vi "通信并与其他模块交互 (子VI).vi"() -> ()   [LabVIEW 2016, in "质控单元.lvlib"]
uses:
  <vilib>/Plasmionique/MB Master/MB_Master_TCP/MB_Master_TCP.lvclass
  D:/Program Files (x86)/National Instruments/LabVIEW 2016/vi.lib/Plasmionique/MB Master/MB_Master/MB_Master.lvclass
  <vilib>/Plasmionique/MB Master/MB_Master/MB_Master.lvclass
  <vilib>/Plasmionique/MB Master/MB Master.lvlib
  <vilib>/Utility/config.llb/NI_LVConfig.lvlib
panel:
  out "CODCr测量状态":u16[](array[numeric])
  out "CODMn测量状态":u16[](array[numeric])
  out "总氮测量状态":u16[](array[numeric])
  out "总磷测量状态":u16[](array[numeric])
  out "氨氮测量状态":u16[](array[numeric])
  out "通讯状态":bool
  out "待处理插入数量":i32
  out "元素":cluster{"命令":string}[](array[cluster])
  out "队列中元素数量":i32
  in  "starting address 6":u16
  in  "values 6":u16[](array[numeric])
  in  "starting address 5":u16
  in  "values 5":u16[](array[numeric])
  in  "starting address 4":u16
  in  "values 4":u16[](array[numeric])
  in  "starting address 3":u16
  in  "values 3":u16[](array[numeric])
  in  "starting address 2":u16
  in  "values 2":u16[](array[numeric])
  in  "values":u16[](array[numeric])
  in  "starting address":u16
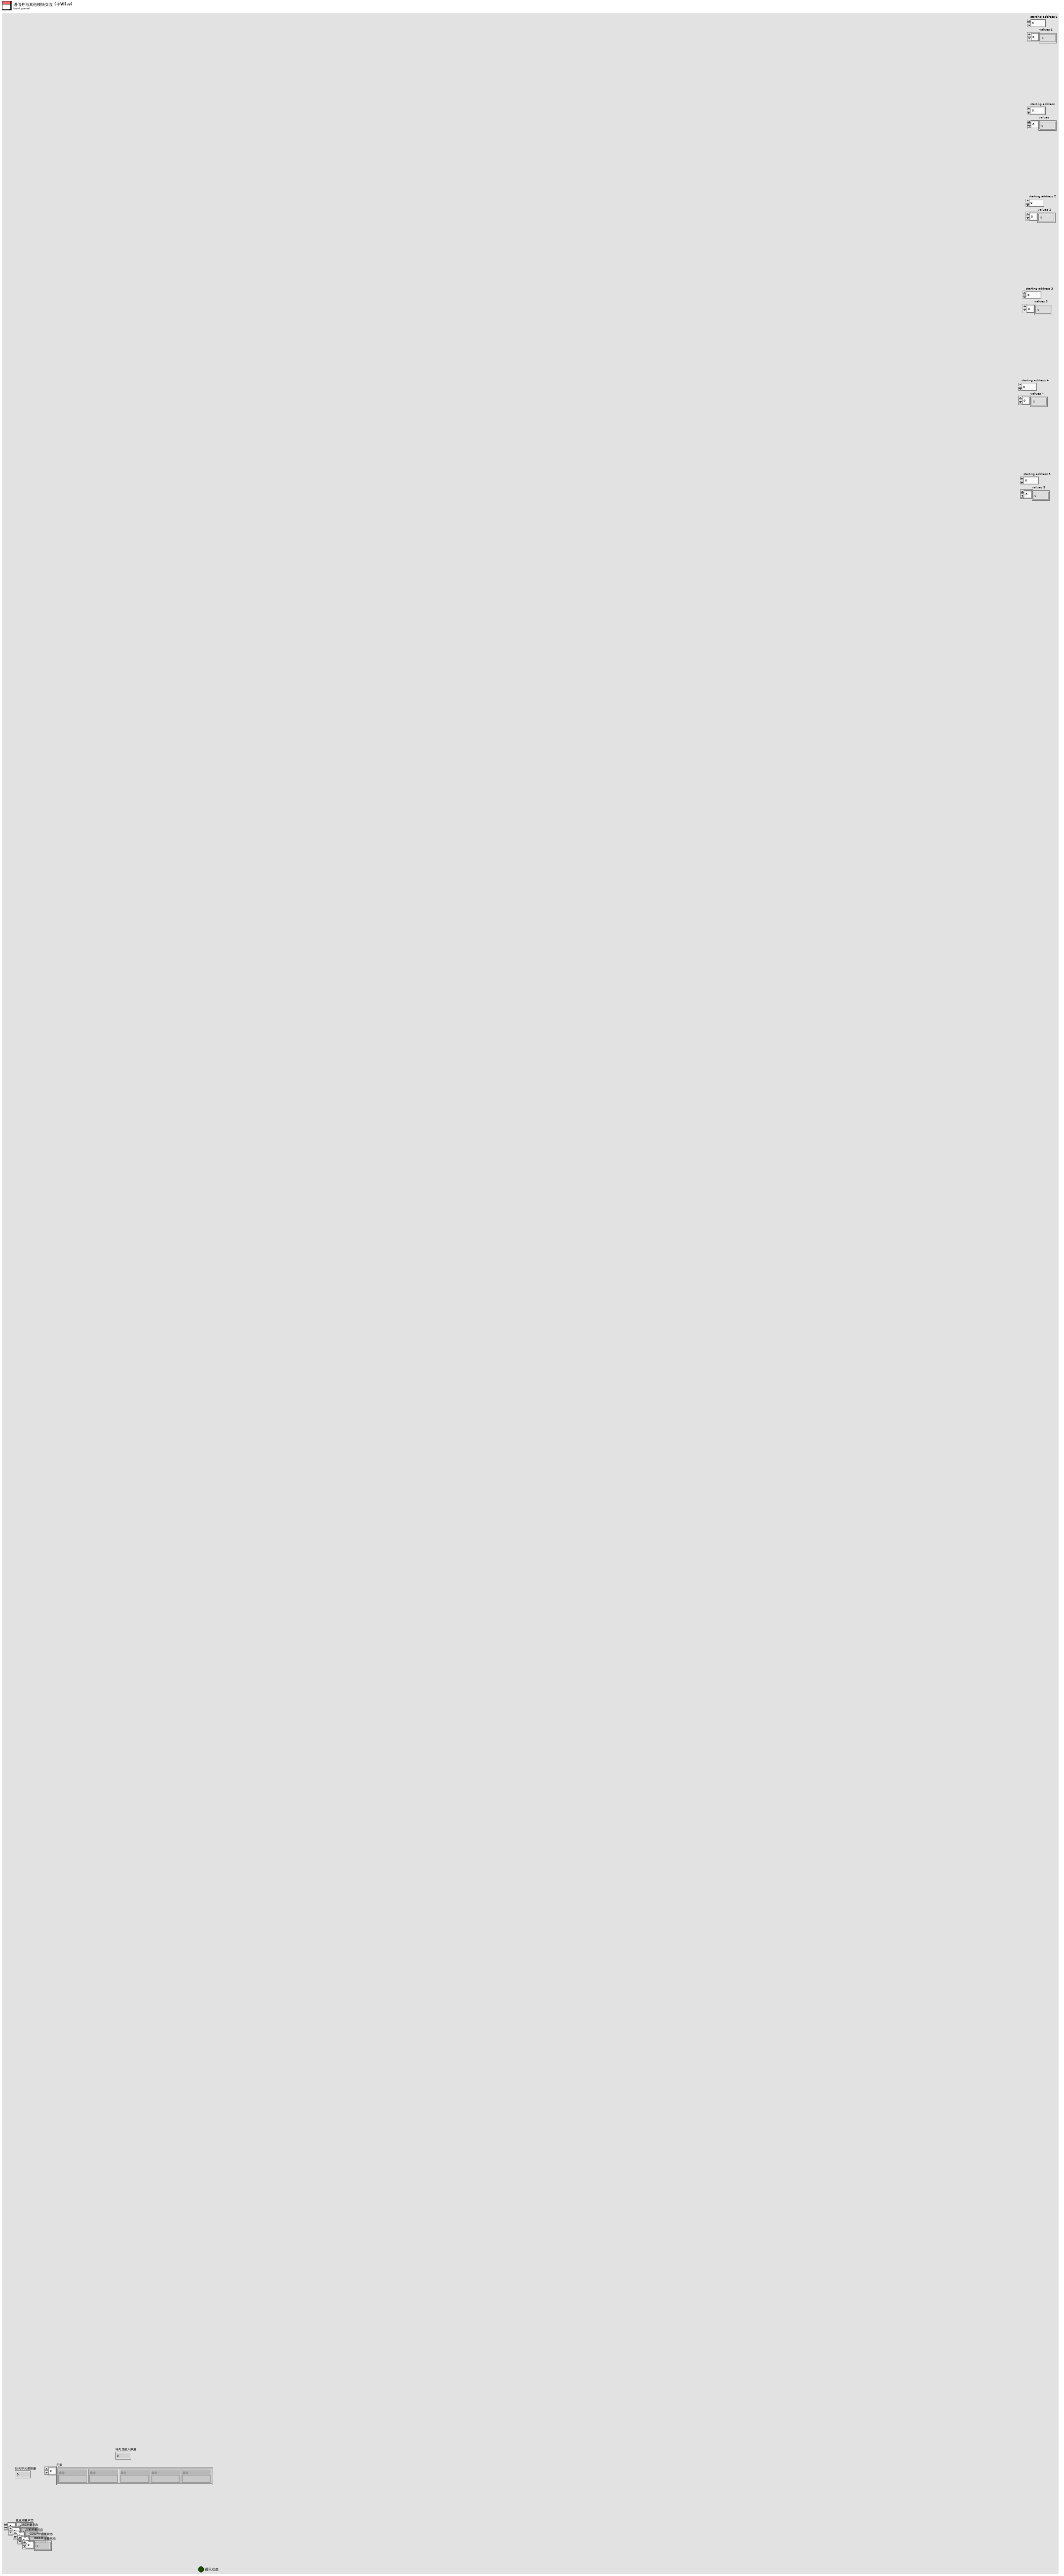
[diagram p1: front panel]
types:
  T1 = typedef "NI_LVConfig.lvlib/Config Data RefNum.ctl" = refnum<k1>
  T2 = cluster{"因子编码":u32, "单位":u16, "标样参考值":sgl, "水样数据时间":timestamp, "水样实测值":sgl, "水样数据标识":string, "标样数据时间":timestamp, "标样实测值":sgl, "标样数据标识":string, "空白数据时间":timestamp, "空白实测值":sgl, "空白数据标识":string, "零点核查数据时间":timestamp, "零点核查实测值":sgl, "零点核查数据标识":string, "跨度核查数据时间":timestamp, "跨度核查实测值":sgl, "跨度核查数据标识":string, "加标回收数据时间":timestamp, "加标回收实测值":sgl, "加标回收数据标识":string, "平行样数据时间":timestamp, "平行样实测值":sgl, "平行样数据标识":string}
  T3 = cluster{"系统时间":timestamp, "工作状态":enum16{"空闲", "水样测试", "标样核查", "零点核查", "跨度核查", "空白测试", "平行样测试", "加标回收", "空白校准", "标样校准", "初始化（清洗）"}, "测量模式":enum16{"待机", "连续模式", "周期模式", "定点模式", "受控模式", "手动模式"}, "告警代码":enum16{"无告警", "缺试剂告警", "缺水样告警", "缺蒸馏水告警", "缺标液告警", "仪表漏液告警", "标定异常告警", "超量程告警", "加热异常", "低试剂预警", "超上限告警", "超下限告警", "仪表内部其他异常", "滴定异常告警", "电极异常告警", "量程切换告警", "参数设置告警", "PH电极电位异常", "电导率电极异常", "浊度光度异常", "溶解氧电极异常", "溶解氧光强异常", "温度异常告警", "PH异常告警", "溶解氧异常告警", "电导率异常告警", "浊度异常告警", "叶绿素异常告警", "藻密度异常告警", "蓝绿藻异常告警", "ORP异常告警", "氨氮异常告警", "清洁刷异常告警", "SD卡异常告警", "蓝牙异常告警", "Wifi异常告警", "流程异常告警"}, "故障代码":enum16{"无故障", "电机故障", "温度故障", "通讯故障", "滴定故障"}, "日志代码":u16, "软件版本":u16, "F0":sgl, "F1":sgl, "F2":sgl, "F3":sgl, "T":sgl, "H":sgl, "id":u16, "flowid":u16, "量程":u16, "总磷控温温度1":sgl, "营养盐控温温度2":sgl, "ADC":sgl}
  T4 = cluster{"Registers[0]":u16, "Registers[1]":u16, "Registers[2]":u16, "Registers[3]":u16, "Registers[4]":u16, "Registers[5]":u16, "Registers[6]":u16, "Registers[7]":u16, "Registers[8]":u16, "Registers[9]":u16, "Registers[10]":u16, "Registers[11]":u16, "Registers[12]":u16, "Registers[13]":u16, "Registers[14]":u16, "Registers[15]":u16, "Registers[16]":u16, "Registers[17]":u16, "Registers[18]":u16, "Registers[19]":u16, "Registers[20]":u16, "Registers[21]":u16, "Registers[22]":u16, "Registers[23]":u16, "Registers[24]":u16, "Registers[25]":u16, "Registers[26]":u16, "Registers[27]":u16, "Registers[28]":u16, "Registers[29]":u16, "Registers[30]":u16, "Registers[31]":u16, "Registers[32]":u16, "Registers[33]":u16, "Registers[34]":u16, "Registers[35]":u16, "Registers[36]":u16, "Registers[37]":u16, "Registers[38]":u16, "Registers[39]":u16, "Registers[40]":u16, "Registers[41]":u16, "Registers[42]":u16, "Registers[43]":u16, "Registers[44]":u16, "Registers[45]":u16, "Registers[46]":u16, "Registers[47]":u16, "Registers[48]":u16, "Registers[49]":u16, "Registers[50]":u16, "Registers[51]":u16, "Registers[52]":u16, "Registers[53]":u16, "Registers[54]":u16, "Registers[55]":u16, "Registers[56]":u16}
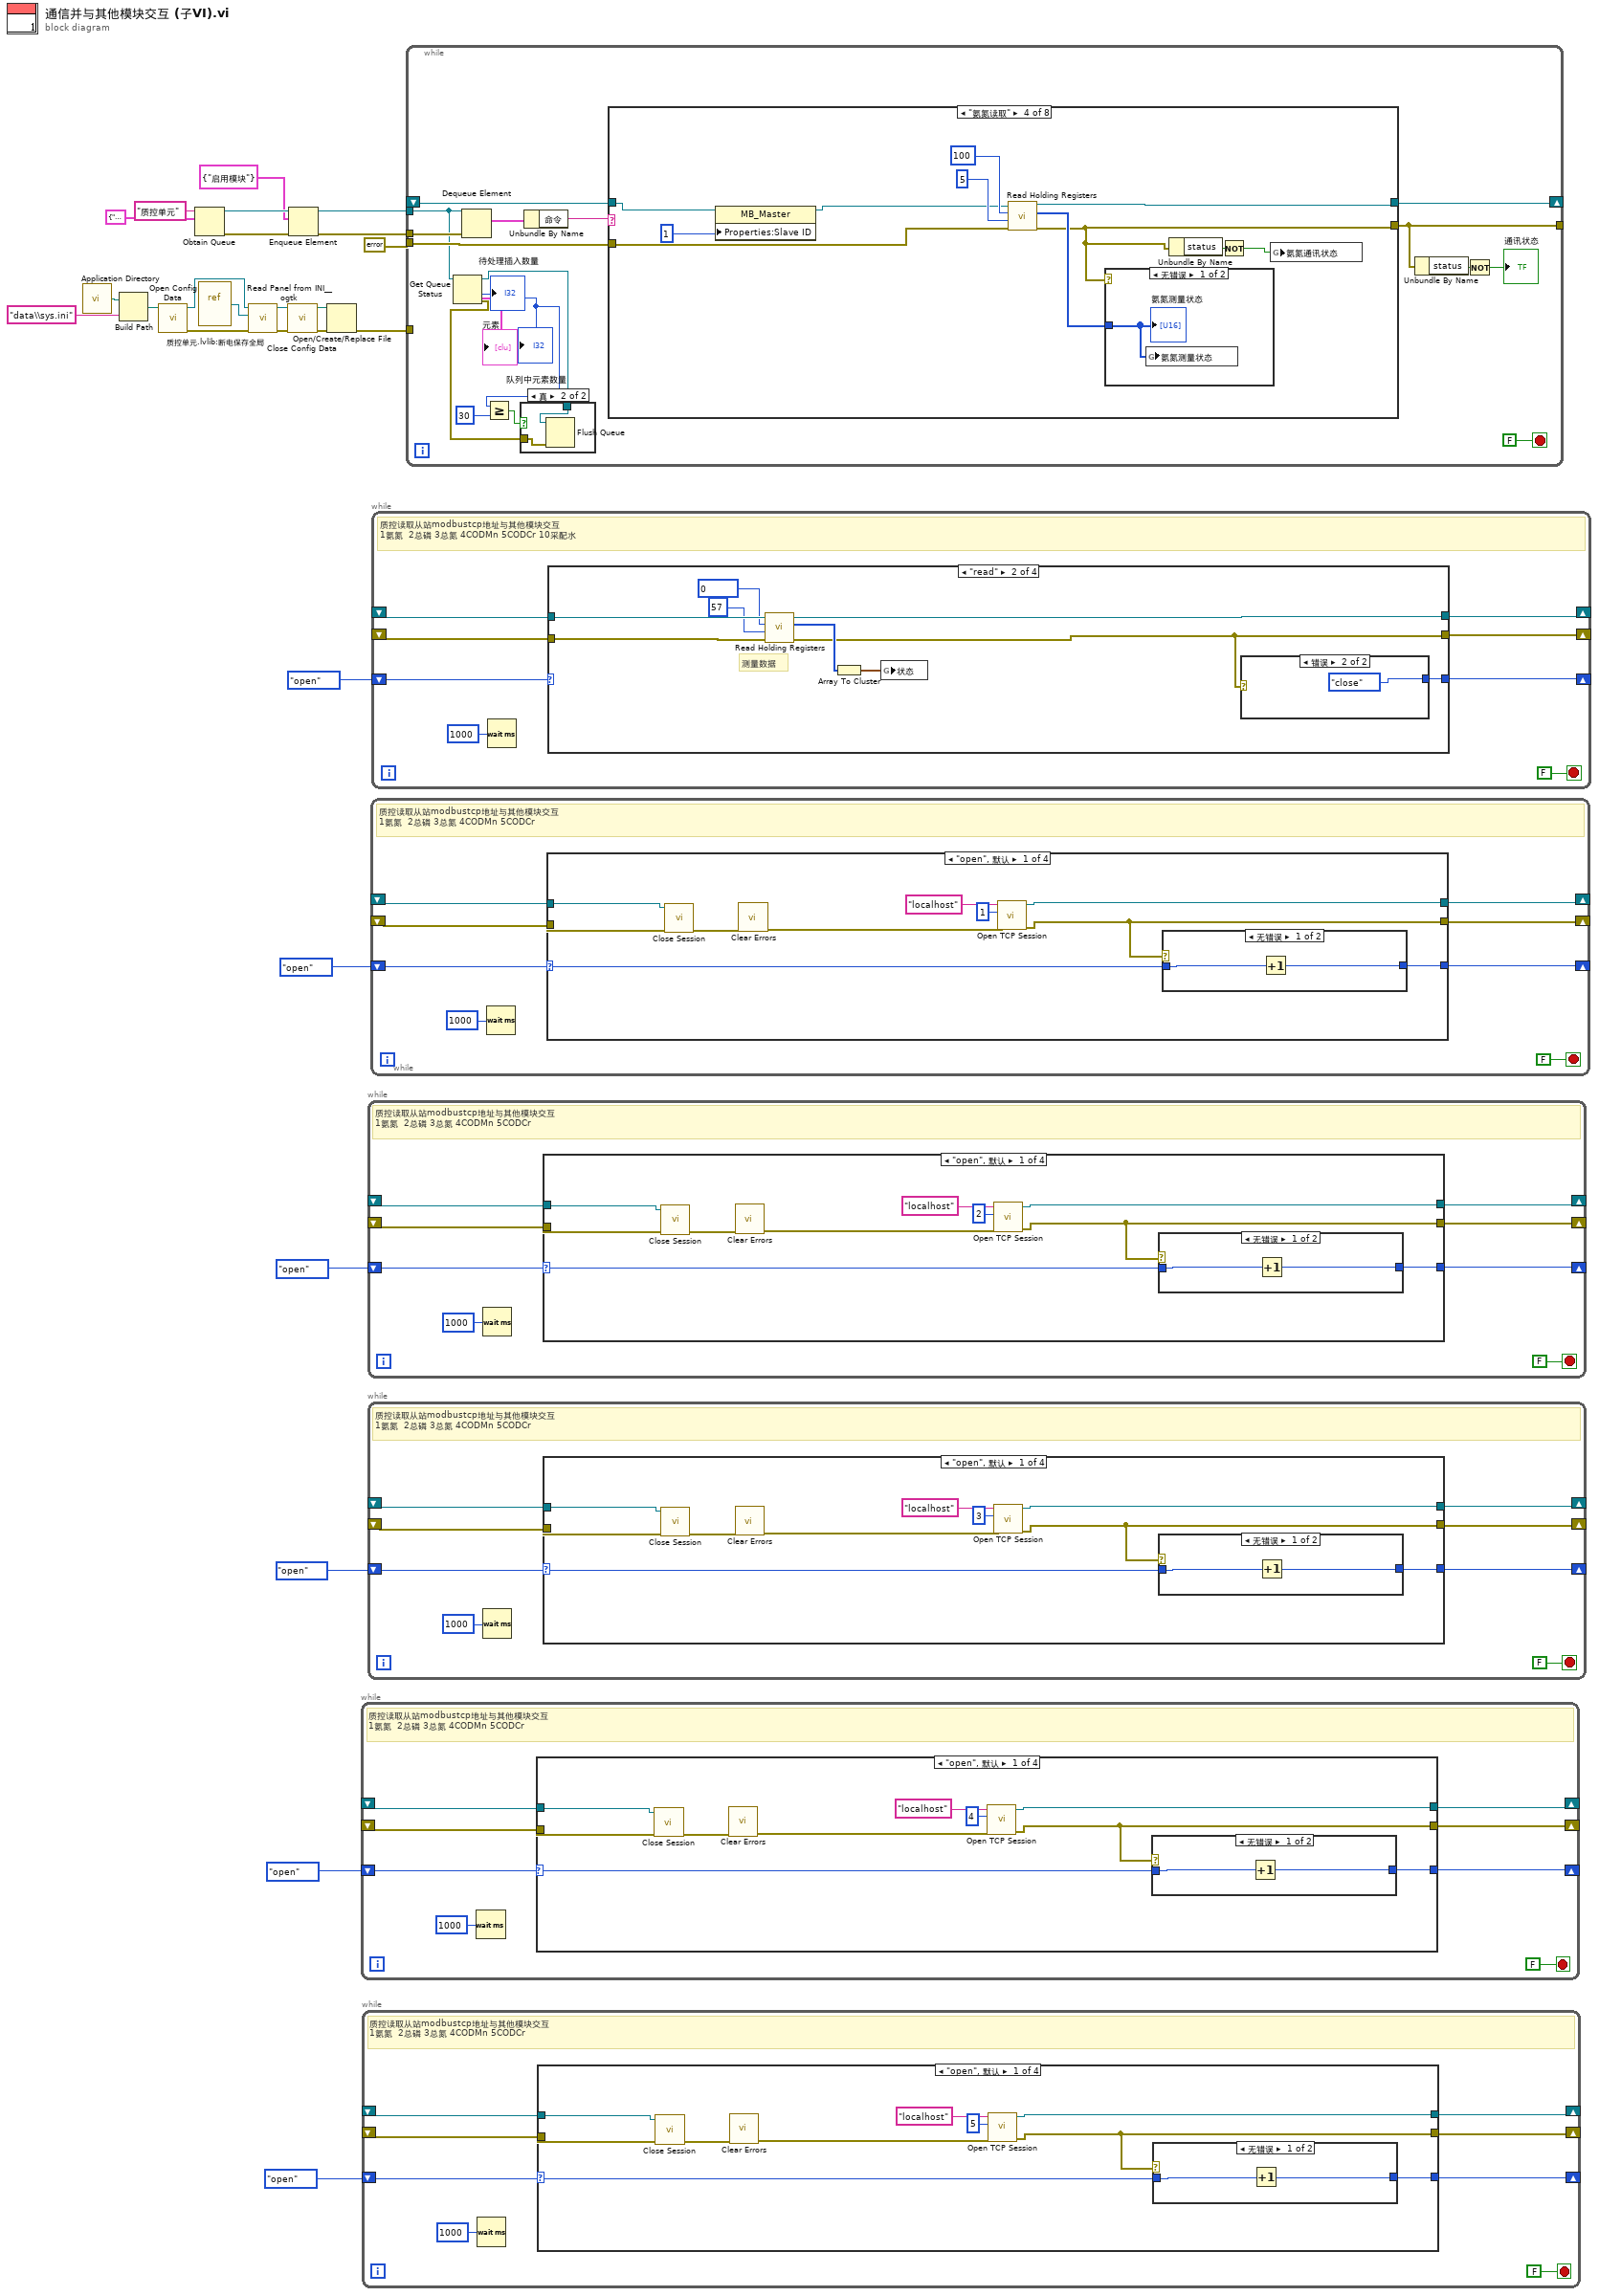
[diagram p0: block diagram]
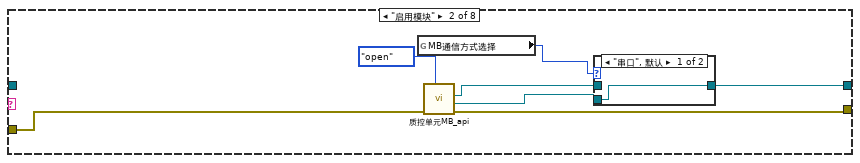
[diagram p4: hidden frame]
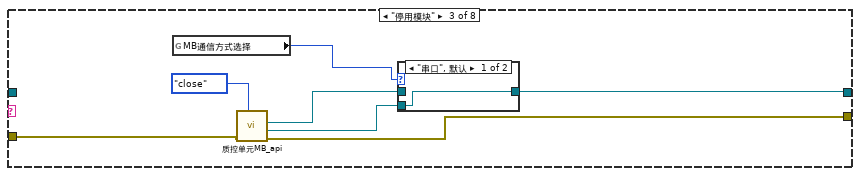
[diagram p6: hidden frame]
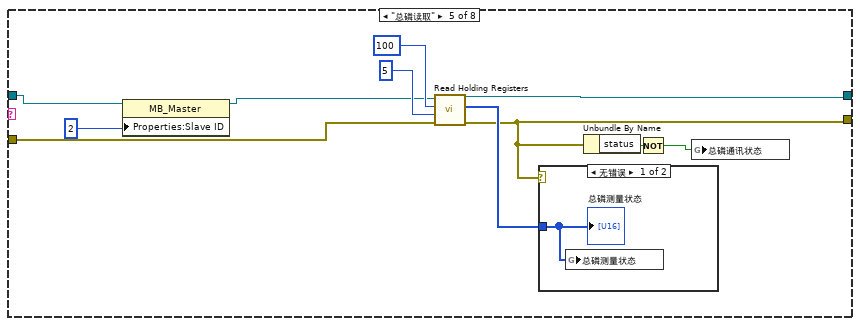
[diagram p9: hidden frame]
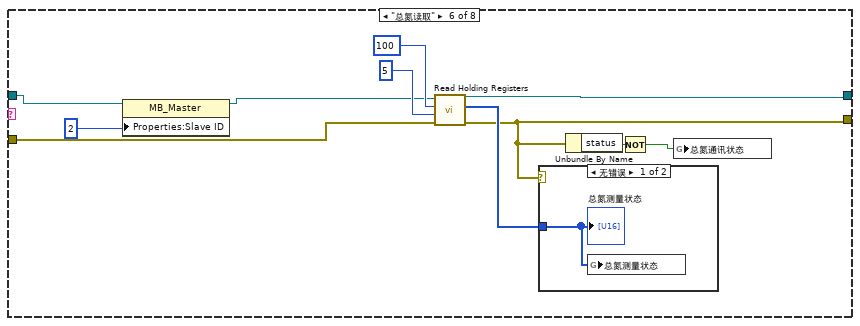
[diagram p11: hidden frame]
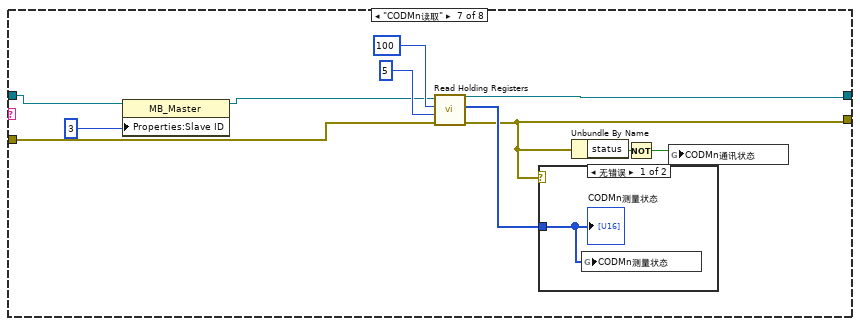
[diagram p13: hidden frame]
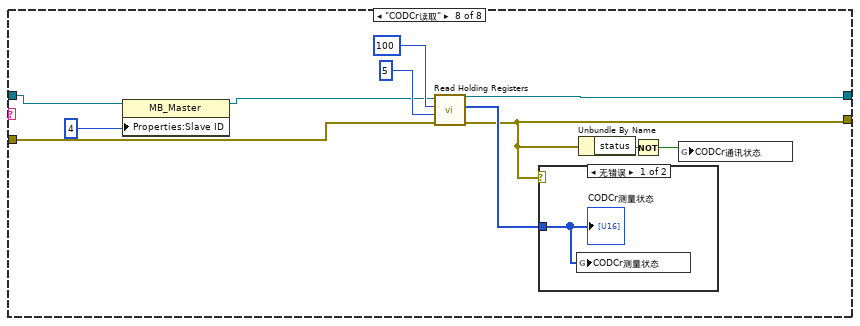
[diagram p15: hidden frame]
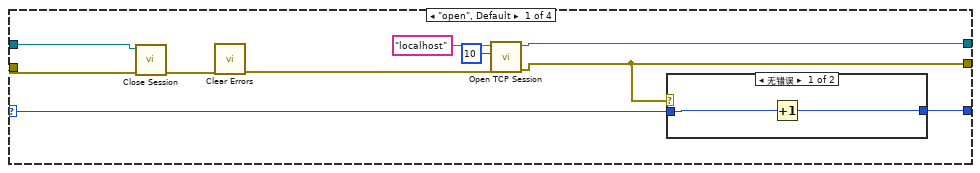
[diagram p17: hidden frame]
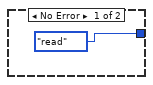
[diagram p19: hidden frame]
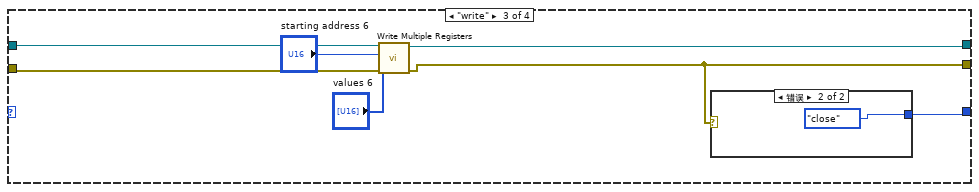
[diagram p20: hidden frame]
diagram:
  n1 = call <vilib>:"Application Directory.vi"() -> ("Application Directory"=w13:path)
  n2 = Build Path(base path=w13, name or relative path="data\\sys.ini" ("名称或相对路径")) -> (appended path=w11:path)
  n3 = call <vilib>:"Open Config Data.vi"("configuration file path"=w11) -> ("error out"=w7:errorcluster, "refnum"=w10:T1)  [unwired: 8 in, 1 out]
  n4 = Obtain Queue(name (unnamed)="质控单元" ("名称（未命名）"), element data type=cluster{"命令":string} {"命令"="启用模块"} ("元素")) -> (queue out=w16:refnum<queue>, error out=w15:errorcluster)  [unwired: 3 in, 1 out]
  n5 = vi-ref "质控单元.lvlib:断电保存全局.vi"() -> (w9:refnum<vi>)
  n6 = call <userlib>:"Read Panel from INI__ogtk.vi"("error in (no error)"=w7, "VI ref"=w9, "refnum"=w10) -> ("error out"=w6:errorcluster, "refnum out"=w8:T1)  [unwired: 7 in]
  n7 = call <vilib>:"Close Config Data.vi"("error in (no error)"=w6, "refnum"=w8) -> ("error out"=w5:errorcluster, "file path"=w4:path)  [unwired: 8 in]
  n8 = Enqueue Element(queue=w16, element=cluster{"命令":string} {"命令"="启用模块"} ("元素"), error in (no error)=w15) -> (queue out=w2:refnum<queue>, error out=w1:errorcluster)  [unwired: 1 in, 1 out]
  n9 = Open/Create/Replace File(file path (use dialog)=w4, error in=w5) -> (error out=w3:errorcluster)  [unwired: 4 in, 2 out]
  n10 = while {
    shift-right: [w31] -> _
    shift-left: _ -> [w33]
    shift-right: [w30] -> _
    shift-left: _ -> [w32]
    shift-right: [w27] -> _
    shift-left: enum16{"open", "read", "write", "close"}."open" -> [w28]
    stop <- FALSE stop-if-true
    # "质控读取从站modbustcp地址与其他模块交互\n1氨氮  2总磷 3总氮 4CODMn 5CODCr"
    n11 = Wait (ms)(milliseconds to wait=u32 1000 ("等待时间（毫秒）")) -> ()  [unwired: 1 out]
    n12 = case shown="\"open\", 默认" w28 {
      selector: w28 -> [w35 _ _ _]
      tunnel: w33 -> [w40 w71 w79 w87]
      tunnel: w32 -> [w39 w68 w78 w86]
      tunnel: [w41 w66 w77 w87] -> w31
      tunnel: [w36 w65 w76 w84] -> w30
      tunnel: [w34 w67 w80 enum16{"open", "read", "write", "close"}."open"] -> w27
      frame "open", Default {
        n13 = call-dynamic "Close Session.vi"("error in (no error)"=w39, "MB session in"=w40) -> ("error out"=w38:errorcluster)  [unwired: 9 in]
        n14 = call <vilib>:"Clear Errors.vi"("error in (no error)"=w38) -> ("error out"=w37:errorcluster)  [unwired: 5 in, 1 out]
        n15 = call <vilib>:"Open TCP Session.vi"("error in (no error)"=w37, "Port (502)"=u16 4, "IP Address"="localhost") -> ("error out"=w36:errorcluster, "MB_TCP session"=w41:refnum<class "MB_Master_TCP.lvclass">)  [unwired: 7 in]
        n16 = case shown="无错误" w36 {
          tunnel: w35 -> [w45 w46]
          tunnel: [w44 w46] -> w34
          frame No Error {
            n17 = Increment(x=w45) -> (x+1=w44:enum16{"open", "read", "write", "close"})
          }
          frame Error {
          }
        }
      }
      frame "read" {
        # "测量数据"
        n18 = call <vilib>:"Read Holding Registers.vi"("error in (no error)"=w68, "quantity"=u16 30, "starting address"=u16 0, "MB session in"=w71) -> ("error out"=w65:errorcluster, "Registers"=w64:u16[], "MB session out"=w66:refnum<class "MB_Master.lvclass">)  [unwired: 5 in]
        n19 = Index Array(array=w64) -> (element #1=w63:u16, element #2=w62:u16, element #3=w61:u16, element #4=w57:u16, element #5=w56:u16, element #6=w55:u16, element #7=w54:u16, element #8=w52:u16, element #9=w51:u16, element #10=w50:u16)  [unwired: 10 in]
        n20 = Build Array(w62, w61) -> (w60:u16[])
        n21 = Build Array(w56, w55, w54, w52, w51, w50) -> (w53:u16[])
        n22 = call "HexToDate.vi"("数组"=w53) -> ("DATE"=w49:timestamp[])  [unwired: 10 in]
        n23 = call "HexToCDABFloat.vi"("数组"=w60) -> ("FLOAT"=w59:sgl[])  [unwired: 10 in]
        n24 = Index Array(array=w49) -> (element #1=w48:timestamp, element #2=w47:timestamp)  [unwired: 2 in]
        n25 = Index Array(array=w59) -> (element=w58:sgl)  [unwired: 1 in]
        n26 = global write "与CODMn交互全局.vi" "COD浓度（mg/L)"(w58) -> ()
        n27 = global write "与CODMn交互全局.vi" "加标回收启动时间"(w48) -> ()
        n28 = global write "与CODMn交互全局.vi" "CODMn工作状态"(w63) -> ()
        n29 = global write "与CODMn交互全局.vi" "水样启动时间"(w47) -> ()
        n30 = global write "与CODMn交互全局.vi" "多列列表框"(w57) -> ()
        n31 = case shown="错误" w65 {
          tunnel: [enum16{"open", "read", "write", "close"}."read" enum16{"open", "read", "write", "close"}."close"] -> w67
          frame No Error {
          }
          frame Error {
          }
        }
      }
      frame "write" {
        n32 = call <vilib>:"Write Multiple Registers.vi"("error in (no error)"=w78, "values"="values 4", "starting address"="starting address 4", "MB session in"=w79) -> ("error out"=w76:errorcluster, "MB session out"=w77:refnum<class "MB_Master.lvclass">)  [unwired: 6 in]
        n33 = case shown="错误" w76 {
          tunnel: [enum16{"open", "read", "write", "close"}."read" enum16{"open", "read", "write", "close"}."close"] -> w80
          frame No Error {
          }
          frame Error {
          }
        }
      }
      frame "close" {
        n34 = call-dynamic "Close Session.vi"("error in (no error)"=w86, "MB session in"=w87) -> ("error out"=w85:errorcluster)  [unwired: 9 in]
        n35 = call <vilib>:"Clear Errors.vi"("error in (no error)"=w85) -> ("error out"=w84:errorcluster)  [unwired: 5 in, 1 out]
      }
    }
  }
  n36 = while {
    shift-right: [w93] -> _
    shift-left: _ -> [w95]
    shift-right: [w92] -> _
    shift-left: _ -> [w94]
    shift-right: [w89] -> _
    shift-left: enum16{"open", "read", "write", "close"}."open" -> [w90]
    stop <- FALSE stop-if-true
    # "质控读取从站modbustcp地址与其他模块交互\n1氨氮  2总磷 3总氮 4CODMn 5CODCr"
    n37 = Wait (ms)(milliseconds to wait=u32 1000 ("等待时间（毫秒）")) -> ()  [unwired: 1 out]
    n38 = case shown="\"open\", 默认" w90 {
      selector: w90 -> [w97 _ _ _]
      tunnel: w95 -> [w102 w123 w131 w139]
      tunnel: w94 -> [w101 w120 w130 w138]
      tunnel: [w103 w114 w129 w139] -> w93
      tunnel: [w98 w113 w128 w136] -> w92
      tunnel: [w96 w119 w132 enum16{"open", "read", "write", "close"}."open"] -> w89
      frame "open", Default {
        n39 = call-dynamic "Close Session.vi"("error in (no error)"=w101, "MB session in"=w102) -> ("error out"=w100:errorcluster)  [unwired: 9 in]
        n40 = call <vilib>:"Clear Errors.vi"("error in (no error)"=w100) -> ("error out"=w99:errorcluster)  [unwired: 5 in, 1 out]
        n41 = call <vilib>:"Open TCP Session.vi"("error in (no error)"=w99, "Port (502)"=u16 5, "IP Address"="localhost") -> ("error out"=w98:errorcluster, "MB_TCP session"=w103:refnum<class "MB_Master_TCP.lvclass">)  [unwired: 7 in]
        n42 = case shown="无错误" w98 {
          tunnel: w97 -> [w107 w108]
          tunnel: [w106 w108] -> w96
          frame No Error {
            n43 = Increment(x=w107) -> (x+1=w106:enum16{"open", "read", "write", "close"})
          }
          frame Error {
          }
        }
      }
      frame "read" {
        # "状态告警"
        # "测量数据"
        n44 = call <vilib>:"Read Holding Registers.vi"("error in (no error)"=w120, "quantity"=u16 83, "starting address"=u16 4096, "MB session in"=w123) -> ("error out"=w115:errorcluster, "Registers"=w112:u16[], "MB session out"=w116:refnum<class "MB_Master.lvclass">)  [unwired: 5 in]
        n45 = call "交互测量数据区解析.vi"("数组"=w112) -> ("测量数据区"=w110:T2)  [unwired: 10 in]
        n46 = global write "与CODCr交互全局.vi" "CODCr测量数据区"(w110) -> ()
        n47 = call <vilib>:"Read Holding Registers.vi"("error in (no error)"=w115, "quantity"=u16 24, "starting address"=u16 4224, "MB session in"=w116) -> ("error out"=w113:errorcluster, "Registers"=w111:u16[], "MB session out"=w114:refnum<class "MB_Master.lvclass">)  [unwired: 5 in]
        n48 = call "交互状态告警区解析.vi"("数组"=w111) -> ("状态告警区"=w109:T3)  [unwired: 10 in]
        n49 = global write "与CODCr交互全局.vi" "CODCr状态告警区"(w109) -> ()
        n50 = case shown="错误" w113 {
          tunnel: [enum16{"open", "read", "write", "close"}."read" enum16{"open", "read", "write", "close"}."close"] -> w119
          frame No Error {
          }
          frame Error {
          }
        }
      }
      frame "write" {
        n51 = call <vilib>:"Write Multiple Registers.vi"("error in (no error)"=w130, "values"="values 5", "starting address"="starting address 5", "MB session in"=w131) -> ("error out"=w128:errorcluster, "MB session out"=w129:refnum<class "MB_Master.lvclass">)  [unwired: 6 in]
        n52 = case shown="错误" w128 {
          tunnel: [enum16{"open", "read", "write", "close"}."read" enum16{"open", "read", "write", "close"}."close"] -> w132
          frame No Error {
          }
          frame Error {
          }
        }
      }
      frame "close" {
        n53 = call-dynamic "Close Session.vi"("error in (no error)"=w138, "MB session in"=w139) -> ("error out"=w137:errorcluster)  [unwired: 9 in]
        n54 = call <vilib>:"Clear Errors.vi"("error in (no error)"=w137) -> ("error out"=w136:errorcluster)  [unwired: 5 in, 1 out]
      }
    }
  }
  n55 = while {
    shift-right: [w145] -> _
    shift-left: _ -> [w147]
    shift-right: [w144] -> _
    shift-left: _ -> [w146]
    shift-right: [w141] -> _
    shift-left: enum16{"open", "read", "write", "close"}."open" -> [w142]
    stop <- FALSE stop-if-true
    # "质控读取从站modbustcp地址与其他模块交互\n1氨氮  2总磷 3总氮 4CODMn 5CODCr"
    n56 = Wait (ms)(milliseconds to wait=u32 1000 ("等待时间（毫秒）")) -> ()  [unwired: 1 out]
    n57 = case shown="\"open\", 默认" w142 {
      selector: w142 -> [w149 _ _ _]
      tunnel: w147 -> [w154 w175 w183 w191]
      tunnel: w146 -> [w153 w172 w182 w190]
      tunnel: [w155 w166 w181 w191] -> w145
      tunnel: [w150 w165 w180 w188] -> w144
      tunnel: [w148 w171 w184 enum16{"open", "read", "write", "close"}."open"] -> w141
      frame "open", Default {
        n58 = call-dynamic "Close Session.vi"("error in (no error)"=w153, "MB session in"=w154) -> ("error out"=w152:errorcluster)  [unwired: 9 in]
        n59 = call <vilib>:"Clear Errors.vi"("error in (no error)"=w152) -> ("error out"=w151:errorcluster)  [unwired: 5 in, 1 out]
        n60 = call <vilib>:"Open TCP Session.vi"("error in (no error)"=w151, "Port (502)"=u16 2, "IP Address"="localhost") -> ("error out"=w150:errorcluster, "MB_TCP session"=w155:refnum<class "MB_Master_TCP.lvclass">)  [unwired: 7 in]
        n61 = case shown="无错误" w150 {
          tunnel: w149 -> [w159 w160]
          tunnel: [w158 w160] -> w148
          frame No Error {
            n62 = Increment(x=w159) -> (x+1=w158:enum16{"open", "read", "write", "close"})
          }
          frame Error {
          }
        }
      }
      frame "read" {
        # "状态告警"
        # "测量数据"
        n63 = call <vilib>:"Read Holding Registers.vi"("error in (no error)"=w172, "quantity"=u16 83, "starting address"=u16 4096, "MB session in"=w175) -> ("error out"=w167:errorcluster, "Registers"=w164:u16[], "MB session out"=w168:refnum<class "MB_Master.lvclass">)  [unwired: 5 in]
        n64 = call "交互测量数据区解析.vi"("数组"=w164) -> ("测量数据区"=w162:T2)  [unwired: 10 in]
        n65 = global write "与总磷交互全局.vi" "总磷测量数据区"(w162) -> ()
        n66 = call <vilib>:"Read Holding Registers.vi"("error in (no error)"=w167, "quantity"=u16 24, "starting address"=u16 4224, "MB session in"=w168) -> ("error out"=w165:errorcluster, "Registers"=w163:u16[], "MB session out"=w166:refnum<class "MB_Master.lvclass">)  [unwired: 5 in]
        n67 = call "交互状态告警区解析.vi"("数组"=w163) -> ("状态告警区"=w161:T3)  [unwired: 10 in]
        n68 = global write "与总磷交互全局.vi" "总磷状态告警区"(w161) -> ()
        n69 = case shown="错误" w165 {
          tunnel: [enum16{"open", "read", "write", "close"}."read" enum16{"open", "read", "write", "close"}."close"] -> w171
          frame No Error {
          }
          frame Error {
          }
        }
      }
      frame "write" {
        n70 = call <vilib>:"Write Multiple Registers.vi"("error in (no error)"=w182, "values"="values 2", "starting address"="starting address 2", "MB session in"=w183) -> ("error out"=w180:errorcluster, "MB session out"=w181:refnum<class "MB_Master.lvclass">)  [unwired: 6 in]
        n71 = case shown="错误" w180 {
          tunnel: [enum16{"open", "read", "write", "close"}."read" enum16{"open", "read", "write", "close"}."close"] -> w184
          frame No Error {
          }
          frame Error {
          }
        }
      }
      frame "close" {
        n72 = call-dynamic "Close Session.vi"("error in (no error)"=w190, "MB session in"=w191) -> ("error out"=w189:errorcluster)  [unwired: 9 in]
        n73 = call <vilib>:"Clear Errors.vi"("error in (no error)"=w189) -> ("error out"=w188:errorcluster)  [unwired: 5 in, 1 out]
      }
    }
  }
  n74 = while {
    shift-right: [w197] -> _
    shift-left: _ -> [w199]
    shift-right: [w196] -> _
    shift-left: _ -> [w198]
    shift-right: [w193] -> _
    shift-left: enum16{"open", "read", "write", "close"}."open" -> [w194]
    stop <- FALSE stop-if-true
    # "质控读取从站modbustcp地址与其他模块交互\n1氨氮  2总磷 3总氮 4CODMn 5CODCr"
    n75 = Wait (ms)(milliseconds to wait=u32 1000 ("等待时间（毫秒）")) -> ()  [unwired: 1 out]
    n76 = case shown="\"open\", 默认" w194 {
      selector: w194 -> [w201 _ _ _]
      tunnel: w199 -> [w206 w227 w235 w243]
      tunnel: w198 -> [w205 w224 w234 w242]
      tunnel: [w207 w218 w233 w243] -> w197
      tunnel: [w202 w217 w232 w240] -> w196
      tunnel: [w200 w223 w236 enum16{"open", "read", "write", "close"}."open"] -> w193
      frame "open", Default {
        n77 = call-dynamic "Close Session.vi"("error in (no error)"=w205, "MB session in"=w206) -> ("error out"=w204:errorcluster)  [unwired: 9 in]
        n78 = call <vilib>:"Clear Errors.vi"("error in (no error)"=w204) -> ("error out"=w203:errorcluster)  [unwired: 5 in, 1 out]
        n79 = call <vilib>:"Open TCP Session.vi"("error in (no error)"=w203, "Port (502)"=u16 3, "IP Address"="localhost") -> ("error out"=w202:errorcluster, "MB_TCP session"=w207:refnum<class "MB_Master_TCP.lvclass">)  [unwired: 7 in]
        n80 = case shown="无错误" w202 {
          tunnel: w201 -> [w211 w212]
          tunnel: [w210 w212] -> w200
          frame No Error {
            n81 = Increment(x=w211) -> (x+1=w210:enum16{"open", "read", "write", "close"})
          }
          frame Error {
          }
        }
      }
      frame "read" {
        # "状态告警"
        # "测量数据"
        n82 = call <vilib>:"Read Holding Registers.vi"("error in (no error)"=w224, "quantity"=u16 83, "starting address"=u16 4096, "MB session in"=w227) -> ("error out"=w219:errorcluster, "Registers"=w216:u16[], "MB session out"=w220:refnum<class "MB_Master.lvclass">)  [unwired: 5 in]
        n83 = call "交互测量数据区解析.vi"("数组"=w216) -> ("测量数据区"=w214:T2)  [unwired: 10 in]
        n84 = global write "与总氮交互全局.vi" "总氮测量数据区"(w214) -> ()
        n85 = call <vilib>:"Read Holding Registers.vi"("error in (no error)"=w219, "quantity"=u16 24, "starting address"=u16 4224, "MB session in"=w220) -> ("error out"=w217:errorcluster, "Registers"=w215:u16[], "MB session out"=w218:refnum<class "MB_Master.lvclass">)  [unwired: 5 in]
        n86 = call "交互状态告警区解析.vi"("数组"=w215) -> ("状态告警区"=w213:T3)  [unwired: 10 in]
        n87 = global write "与总氮交互全局.vi" "总氮状态告警区"(w213) -> ()
        n88 = case shown="错误" w217 {
          tunnel: [enum16{"open", "read", "write", "close"}."read" enum16{"open", "read", "write", "close"}."close"] -> w223
          frame No Error {
          }
          frame Error {
          }
        }
      }
      frame "write" {
        n89 = call <vilib>:"Write Multiple Registers.vi"("error in (no error)"=w234, "values"="values 3", "starting address"="starting address 3", "MB session in"=w235) -> ("error out"=w232:errorcluster, "MB session out"=w233:refnum<class "MB_Master.lvclass">)  [unwired: 6 in]
        n90 = case shown="错误" w232 {
          tunnel: [enum16{"open", "read", "write", "close"}."read" enum16{"open", "read", "write", "close"}."close"] -> w236
          frame No Error {
          }
          frame Error {
          }
        }
      }
      frame "close" {
        n91 = call-dynamic "Close Session.vi"("error in (no error)"=w242, "MB session in"=w243) -> ("error out"=w241:errorcluster)  [unwired: 9 in]
        n92 = call <vilib>:"Clear Errors.vi"("error in (no error)"=w241) -> ("error out"=w240:errorcluster)  [unwired: 5 in, 1 out]
      }
    }
  }
  n93 = while {
    shift-right: [w249] -> _
    shift-left: _ -> [w251]
    shift-right: [w248] -> _
    shift-left: _ -> [w250]
    shift-right: [w245] -> _
    shift-left: enum16{"open", "read", "write", "close"}."open" -> [w246]
    stop <- FALSE stop-if-true
    # "质控读取从站modbustcp地址与其他模块交互\n1氨氮  2总磷 3总氮 4CODMn 5CODCr"
    n94 = Wait (ms)(milliseconds to wait=u32 1000 ("等待时间（毫秒）")) -> ()  [unwired: 1 out]
    n95 = case shown="\"open\", 默认" w246 {
      selector: w246 -> [w253 _ _ _]
      tunnel: w251 -> [w258 w279 w287 w295]
      tunnel: w250 -> [w257 w276 w286 w294]
      tunnel: [w259 w270 w285 w295] -> w249
      tunnel: [w254 w269 w284 w292] -> w248
      tunnel: [w252 w275 w288 enum16{"open", "read", "write", "close"}."open"] -> w245
      frame "open", Default {
        n96 = call-dynamic "Close Session.vi"("error in (no error)"=w257, "MB session in"=w258) -> ("error out"=w256:errorcluster)  [unwired: 9 in]
        n97 = call <vilib>:"Clear Errors.vi"("error in (no error)"=w256) -> ("error out"=w255:errorcluster)  [unwired: 5 in, 1 out]
        n98 = call <vilib>:"Open TCP Session.vi"("error in (no error)"=w255, "Port (502)"=u16 1, "IP Address"="localhost") -> ("error out"=w254:errorcluster, "MB_TCP session"=w259:refnum<class "MB_Master_TCP.lvclass">)  [unwired: 7 in]
        n99 = case shown="无错误" w254 {
          tunnel: w253 -> [w263 w264]
          tunnel: [w262 w264] -> w252
          frame No Error {
            n100 = Increment(x=w263) -> (x+1=w262:enum16{"open", "read", "write", "close"})
          }
          frame Error {
          }
        }
      }
      frame "read" {
        # "状态告警"
        # "测量数据"
        n101 = call <vilib>:"Read Holding Registers.vi"("error in (no error)"=w276, "quantity"=u16 83, "starting address"=u16 4096, "MB session in"=w279) -> ("error out"=w271:errorcluster, "Registers"=w268:u16[], "MB session out"=w272:refnum<class "MB_Master.lvclass">)  [unwired: 5 in]
        n102 = call "交互测量数据区解析.vi"("数组"=w268) -> ("测量数据区"=w267:T2)  [unwired: 10 in]
        n103 = global write "与氨氮交互全局.vi" "氨氮测量数据区"(w267) -> ()
        n104 = call <vilib>:"Read Holding Registers.vi"("error in (no error)"=w271, "quantity"=u16 24, "starting address"=u16 4224, "MB session in"=w272) -> ("error out"=w269:errorcluster, "Registers"=w266:u16[], "MB session out"=w270:refnum<class "MB_Master.lvclass">)  [unwired: 5 in]
        n105 = call "交互状态告警区解析.vi"("数组"=w266) -> ("状态告警区"=w265:T3)  [unwired: 10 in]
        n106 = global write "与氨氮交互全局.vi" "氨氮状态告警区"(w265) -> ()
        n107 = case shown="错误" w269 {
          tunnel: [enum16{"open", "read", "write", "close"}."read" enum16{"open", "read", "write", "close"}."close"] -> w275
          frame No Error {
          }
          frame Error {
          }
        }
      }
      frame "write" {
        n108 = call <vilib>:"Write Multiple Registers.vi"("error in (no error)"=w286, "values"="values", "starting address"="starting address", "MB session in"=w287) -> ("error out"=w284:errorcluster, "MB session out"=w285:refnum<class "MB_Master.lvclass">)  [unwired: 6 in]
        n109 = case shown="错误" w284 {
          tunnel: [enum16{"open", "read", "write", "close"}."read" enum16{"open", "read", "write", "close"}."close"] -> w288
          frame No Error {
          }
          frame Error {
          }
        }
      }
      frame "close" {
        n110 = call-dynamic "Close Session.vi"("error in (no error)"=w294, "MB session in"=w295) -> ("error out"=w293:errorcluster)  [unwired: 9 in]
        n111 = call <vilib>:"Clear Errors.vi"("error in (no error)"=w293) -> ("error out"=w292:errorcluster)  [unwired: 5 in, 1 out]
      }
    }
  }
  n112 = while {
    shift-right: [w301] -> _
    shift-left: _ -> [w303]
    shift-right: [w300] -> _
    shift-left: _ -> [w302]
    shift-right: [w297] -> _
    shift-left: enum16{"open", "read", "write", "close"}."open" -> [w298]
    stop <- FALSE stop-if-true
    # "质控读取从站modbustcp地址与其他模块交互\n1氨氮  2总磷 3总氮 4CODMn 5CODCr 10采配水"
    n113 = Wait (ms)(milliseconds to wait=u32 1000 ("等待时间（毫秒）")) -> ()  [unwired: 1 out]
    n114 = case shown="\"read\"" w298 {
      selector: w298 -> [w305 _ _ _]
      tunnel: w303 -> [w310 w325 w333 w341]
      tunnel: w302 -> [w309 w322 w332 w340]
      tunnel: [w311 w318 w331 w341] -> w301
      tunnel: [w306 w317 w330 w338] -> w300
      tunnel: [w304 w321 w334 enum16{"open", "read", "write", "close"}."open"] -> w297
      frame "open", Default {
        n115 = call-dynamic "Close Session.vi"("error in (no error)"=w309, "MB session in"=w310) -> ("error out"=w308:errorcluster)  [unwired: 9 in]
        n116 = call <vilib>:"Clear Errors.vi"("error in (no error)"=w308) -> ("error out"=w307:errorcluster)  [unwired: 5 in, 1 out]
        n117 = call <vilib>:"Open TCP Session.vi"("error in (no error)"=w307, "Port (502)"=u16 10, "IP Address"="localhost") -> ("error out"=w306:errorcluster, "MB_TCP session"=w311:refnum<class "MB_Master_TCP.lvclass">)  [unwired: 7 in]
        n118 = case shown="无错误" w306 {
          tunnel: w305 -> [w315 w316]
          tunnel: [w314 w316] -> w304
          frame No Error {
            n119 = Increment(x=w315) -> (x+1=w314:enum16{"open", "read", "write", "close"})
          }
          frame Error {
          }
        }
      }
      frame "read" {
        # "测量数据"
        n120 = call <vilib>:"Read Holding Registers.vi"("error in (no error)"=w322, "quantity"=u16 57, "starting address"=u16 0, "MB session in"=w325) -> ("error out"=w317:errorcluster, "Registers"=w320:u16[], "MB session out"=w318:refnum<class "MB_Master.lvclass">)  [unwired: 5 in]
        n121 = Array To Cluster(array=w320) -> (cluster=w319:T4)
        n122 = global write "与采配水交互全局.vi" "状态"(w319) -> ()
        n123 = case shown="错误" w317 {
          tunnel: [enum16{"open", "read", "write", "close"}."read" enum16{"open", "read", "write", "close"}."close"] -> w321
          frame No Error {
          }
          frame Error {
          }
        }
      }
      frame "write" {
        n124 = call <vilib>:"Write Multiple Registers.vi"("error in (no error)"=w332, "values"="values 6", "starting address"="starting address 6", "MB session in"=w333) -> ("error out"=w330:errorcluster, "MB session out"=w331:refnum<class "MB_Master.lvclass">)  [unwired: 6 in]
        n125 = case shown="错误" w330 {
          tunnel: [enum16{"open", "read", "write", "close"}."read" enum16{"open", "read", "write", "close"}."close"] -> w334
          frame No Error {
          }
          frame Error {
          }
        }
      }
      frame "close" {
        n126 = call-dynamic "Close Session.vi"("error in (no error)"=w340, "MB session in"=w341) -> ("error out"=w339:errorcluster)  [unwired: 9 in]
        n127 = call <vilib>:"Clear Errors.vi"("error in (no error)"=w339) -> ("error out"=w338:errorcluster)  [unwired: 5 in, 1 out]
      }
    }
  }
  n128 = while {
    tunnel: w2 -> [w349]
    tunnel: w1 -> [w358]
    tunnel: [w350] -> _
    shift-right: [w354] -> _
    shift-left: _ -> [w353]
    tunnel: errorcluster {"status"=FALSE, "code"=0, "source"=""} ("error out") -> [w352]
    tunnel: w3 -> [_]
    stop <- FALSE stop-if-true
    n129 = Get Queue Status(queue=w349) -> (queue out=w343:refnum<queue>, # pending insert=→"待处理插入数量":i32, error out=w342:errorcluster, # elements in queue=w346:i32, elements=→"元素":cluster{"命令":string}[])  [unwired: 2 in, 3 out]
    "队列中元素数量" <- w346
    n130 = Dequeue Element(queue=w349, error in (no error)=w358) -> (element=w357:cluster{"命令":string})  [unwired: 1 in, 3 out]
    n131 = Greater Or Equal?(x=w346, y=30) -> (x >= y?=w344:bool)
    n132 = case shown="真" w344 {
      tunnel: w343 -> [_ w361]
      tunnel: w342 -> [_ w360]
      frame False {
      }
      frame True {
        n133 = Flush Queue(queue=w361, error in (no error)=w360) -> ()  [unwired: 3 out]
      }
    }
    n134 = Unbundle By Name(w357) -> ("命令"=w356:string)
    n135 = case shown="\"氨氮读取\"" w356 {
      tunnel: [w363 w365 w375 w388 w400 w412 w424 w436] -> w354
      tunnel: [w362 w370 w377 w383 w394 w406 w418 w430] -> w350
      tunnel: w353 -> [w363 _ _ w386 w398 w410 w422 w434]
      tunnel: w352 -> [w362 w368 w378 w392 w404 w416 w428 w440]
      frame Default {
      }
      frame "启用模块" {
        n136 = global read "断电保存全局.vi" "MB通信方式选择"() -> (w364:enum16{"串口", "TCP"})
        n137 = call "质控单元MB_api.vi"("STEP"=enum16{"open", "read", "write", "close"}."open", "Error in"=w368) -> ("error out"=w370:errorcluster, "MB session out"=w366:refnum<class "MB_Master.lvclass">, "MB_TCP session"=w367:refnum<class "MB_Master_TCP.lvclass">)  [unwired: 6 in, 1 out]
        n138 = case shown="\"串口\", 默认" w364 {
          tunnel: w367 -> [_ w372]
          tunnel: w366 -> [w371 _]
          tunnel: [w371 w372] -> w365
          frame "串口", Default {
          }
          frame "TCP" {
          }
        }
      }
      frame "停用模块" {
        n139 = global read "断电保存全局.vi" "MB通信方式选择"() -> (w373:enum16{"串口", "TCP"})
        n140 = call "质控单元MB_api.vi"("STEP"=enum16{"open", "read", "write", "close"}."close", "Error in"=w378) -> ("error out"=w377:errorcluster, "MB session out"=w376:refnum<class "MB_Master.lvclass">, "MB_TCP session"=w374:refnum<class "MB_Master_TCP.lvclass">)  [unwired: 6 in, 1 out]
        n141 = case shown="\"串口\", 默认" w373 {
          tunnel: w374 -> [_ w381]
          tunnel: w376 -> [w380 _]
          tunnel: [w380 w381] -> w375
          frame "串口", Default {
          }
          frame "TCP" {
          }
        }
      }
      frame "氨氮读取" {
        n142 = property class="MB_Master"(reference=w386, "Properties:Slave ID"=u8 1 ("Slave ID")) -> (reference out=w385:refnum<class "MB_Master.lvclass">)  [unwired: 1 in, 1 out]
        n143 = call <vilib>:"Read Holding Registers.vi"("error in (no error)"=w392, "quantity"=u16 5 ("number of holding registers"), "starting address"=u16 100, "MB session in"=w385) -> ("error out"=w383:errorcluster, "Registers"=w389:u16[], "MB session out"=w388:refnum<class "MB_Master.lvclass">)  [unwired: 5 in]
        n144 = case shown="无错误" w383 {
          tunnel: w389 -> [w393 _]
          frame No Error {
            n145 = global write "质控内部交互全局.vi" "氨氮测量状态"(w393) -> ()
            "氨氮测量状态" <- w393
          }
          frame Error {
          }
        }
        n146 = Unbundle By Name(w383) -> ("status"=w384:bool)
        n147 = Not(x=w384) -> (.not. x?=w382:bool)
        n148 = global write "质控内部交互全局.vi" "氨氮通讯状态"(w382) -> ()
      }
      frame "总磷读取" {
        n149 = property class="MB_Master"(reference=w398, "Properties:Slave ID"=u8 2 ("Slave ID")) -> (reference out=w397:refnum<class "MB_Master.lvclass">)  [unwired: 1 in, 1 out]
        n150 = call <vilib>:"Read Holding Registers.vi"("error in (no error)"=w404, "quantity"=u16 5 ("number of holding registers"), "starting address"=u16 100, "MB session in"=w397) -> ("error out"=w394:errorcluster, "Registers"=w401:u16[], "MB session out"=w400:refnum<class "MB_Master.lvclass">)  [unwired: 5 in]
        n151 = case shown="无错误" w394 {
          tunnel: w401 -> [w405 _]
          frame No Error {
            n152 = global write "质控内部交互全局.vi" "总磷测量状态"(w405) -> ()
            "总磷测量状态" <- w405
          }
          frame Error {
          }
        }
        n153 = Unbundle By Name(w394) -> ("status"=w396:bool)
        n154 = Not(x=w396) -> (.not. x?=w395:bool)
        n155 = global write "质控内部交互全局.vi" "总磷通讯状态"(w395) -> ()
      }
      frame "总氮读取" {
        n156 = property class="MB_Master"(reference=w410, "Properties:Slave ID"=u8 2 ("Slave ID")) -> (reference out=w409:refnum<class "MB_Master.lvclass">)  [unwired: 1 in, 1 out]
        n157 = call <vilib>:"Read Holding Registers.vi"("error in (no error)"=w416, "quantity"=u16 5 ("number of holding registers"), "starting address"=u16 100, "MB session in"=w409) -> ("error out"=w406:errorcluster, "Registers"=w413:u16[], "MB session out"=w412:refnum<class "MB_Master.lvclass">)  [unwired: 5 in]
        n158 = case shown="无错误" w406 {
          tunnel: w413 -> [w417 _]
          frame No Error {
            n159 = global write "质控内部交互全局.vi" "总氮测量状态"(w417) -> ()
            "总氮测量状态" <- w417
          }
          frame Error {
          }
        }
        n160 = Unbundle By Name(w406) -> ("status"=w408:bool)
        n161 = Not(x=w408) -> (.not. x?=w407:bool)
        n162 = global write "质控内部交互全局.vi" "总氮通讯状态"(w407) -> ()
      }
      frame "CODMn读取" {
        n163 = property class="MB_Master"(reference=w422, "Properties:Slave ID"=u8 3 ("Slave ID")) -> (reference out=w421:refnum<class "MB_Master.lvclass">)  [unwired: 1 in, 1 out]
        n164 = call <vilib>:"Read Holding Registers.vi"("error in (no error)"=w428, "quantity"=u16 5 ("number of holding registers"), "starting address"=u16 100, "MB session in"=w421) -> ("error out"=w418:errorcluster, "Registers"=w425:u16[], "MB session out"=w424:refnum<class "MB_Master.lvclass">)  [unwired: 5 in]
        n165 = case shown="无错误" w418 {
          tunnel: w425 -> [w429 _]
          frame No Error {
            n166 = global write "质控内部交互全局.vi" "CODMn测量状态"(w429) -> ()
            "CODMn测量状态" <- w429
          }
          frame Error {
          }
        }
        n167 = Unbundle By Name(w418) -> ("status"=w420:bool)
        n168 = Not(x=w420) -> (.not. x?=w419:bool)
        n169 = global write "质控内部交互全局.vi" "CODMn通讯状态"(w419) -> ()
      }
      frame "CODCr读取" {
        n170 = property class="MB_Master"(reference=w434, "Properties:Slave ID"=u8 4 ("Slave ID")) -> (reference out=w433:refnum<class "MB_Master.lvclass">)  [unwired: 1 in, 1 out]
        n171 = call <vilib>:"Read Holding Registers.vi"("error in (no error)"=w440, "quantity"=u16 5 ("number of holding registers"), "starting address"=u16 100, "MB session in"=w433) -> ("error out"=w430:errorcluster, "Registers"=w437:u16[], "MB session out"=w436:refnum<class "MB_Master.lvclass">)  [unwired: 5 in]
        n172 = case shown="无错误" w430 {
          tunnel: w437 -> [w441 _]
          frame No Error {
            n173 = global write "质控内部交互全局.vi" "CODCr测量状态"(w441) -> ()
            "CODCr测量状态" <- w441
          }
          frame Error {
          }
        }
        n174 = Unbundle By Name(w430) -> ("status"=w432:bool)
        n175 = Not(x=w432) -> (.not. x?=w431:bool)
        n176 = global write "质控内部交互全局.vi" "CODCr通讯状态"(w431) -> ()
      }
    }
    n177 = Unbundle By Name(w350) -> ("status"=w355:bool)
    n178 = Not(x=w355) -> (.not. x?=→"通讯状态":bool)
  }
